vi "cube rotate left.vi"(8 "error in (no error)":errorcluster, 11 "cube in":T1) -> (0 "error out":errorcluster, 3 "cube out":T1)   [LabVIEW 2011]
uses:
  Typedef/cube.ctl
  Typedef/face.ctl
  Typedef/face rotate direction.ctl
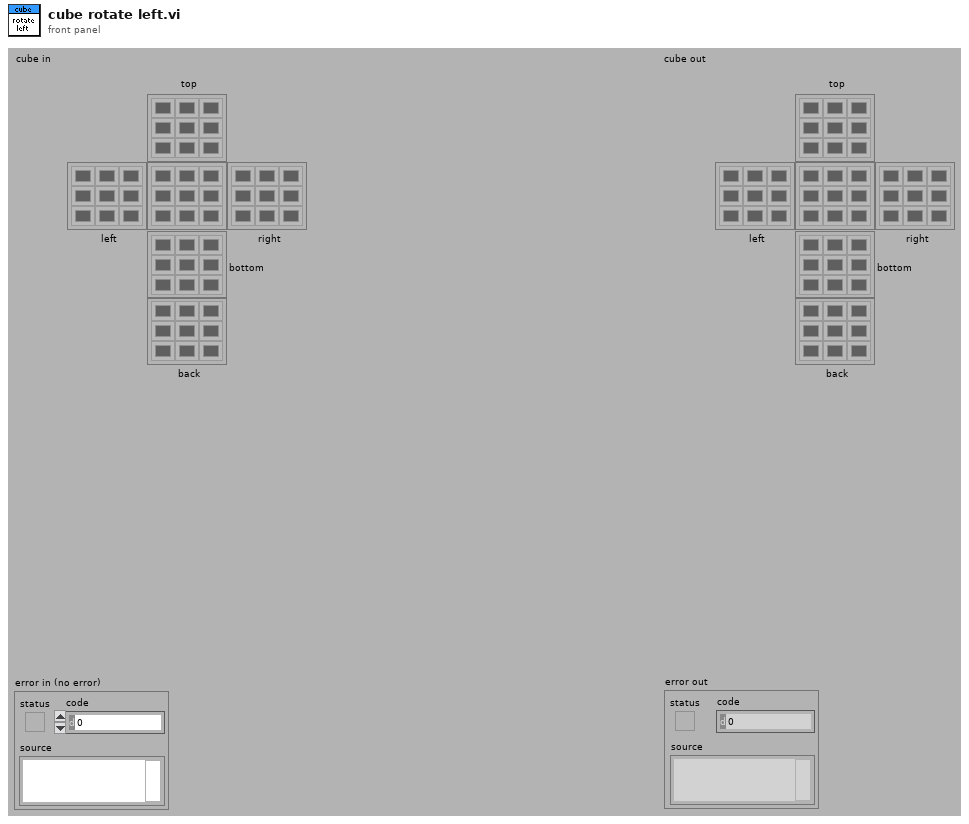
[diagram p1: front panel]
types:
  T1 = typedef "cube.ctl" = cluster{"top":T2, "left":T2, "right":T2, "bottom":T2, "back":T2, "front":T2}
  T2 = typedef "face.ctl" = u32[][]
  T3 = typedef "face rotate direction.ctl" = enum16{"+", "-"}
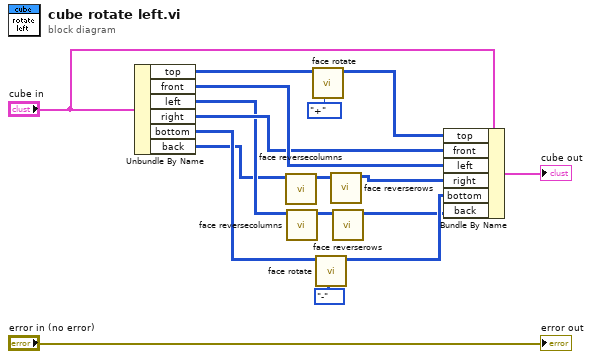
[diagram p0: block diagram]
diagram:
  n1 = Unbundle By Name("cube in") -> ("top"=w12:T2, "front"=w8:T2, "left"=w6:T2, "right"=w7:T2, "bottom"=w10:T2, "back"=w5:T2)
  n2 = call "face reversecolumns.vi"("face in"=w5) -> ("face out"=w4:T2)  [unwired: 9 in, 1 out]
  n3 = call "face reversecolumns.vi"("face in"=w6) -> ("face out"=w2:T2)  [unwired: 9 in, 1 out]
  n4 = call "face rotate.vi"("rotation directon"=face_rotate_direction."+", "face in"=w12) -> ("face out"=w11:T2)  [unwired: 8 in, 1 out]
  n5 = call "face rotate.vi"("rotation directon"=face_rotate_direction."-", "face in"=w10) -> ("face out"=w9:T2)  [unwired: 8 in, 1 out]
  n6 = call "face reverserows.vi"("face in"=w4) -> ("face out"=w3:T2)  [unwired: 9 in, 1 out]
  n7 = call "face reverserows.vi"("face in"=w2) -> ("face out"=w1:T2)  [unwired: 9 in, 1 out]
  n8 = Bundle By Name(cluster="cube in", "top"=w11, "front"=w7, "left"=w8, "right"=w3, "bottom"=w9, "back"=w1) -> (→"cube out":T1)
  "error out" <- "error in (no error)"
